vi "Configure Output Resistance.vi"(0 "VISA resource name":refnum<visa-resource-name>, 1 "List of Source Type":i32[](array[ring])=[1] items=["CURR", "VOLT"], 2 "Shunt Resistance Level (2E+9 Ohm)":dbl=2000000000.0, 3 "Enable Programmable Output (F: Disable)":bool, 5 "Output Channel (0: Channel 1)":i32(ring) items=["Channel 1", "Channel 2"], 7 "Source Mode (1: Voltage)":i32(ring)=1 items=["Current", "Voltage"], 9 "Operation Mode (0: Fixed)":i32(ring) items=["Fixed", "Emulate"], 11 "error in (no error)":errorcluster, 12 "List of Output Data":dbl[](array[numeric])=[0.0, 0.0], 13 "Series Resistance Level (0 Ohm)":dbl) -> (4 "VISA resource name out":refnum<visa-resource-name>, 15 "error out":errorcluster)   [LabVIEW 2023, in "Agilent B2900 Series.lvlib"]
doc: "Configure the output resistance.\n\n<B>Note:</B>\nThis VI is only supported by Agilent models B2961A, B2962A, B2961B and B2962B."
uses:
  Agilent B2900 Series.lvlib
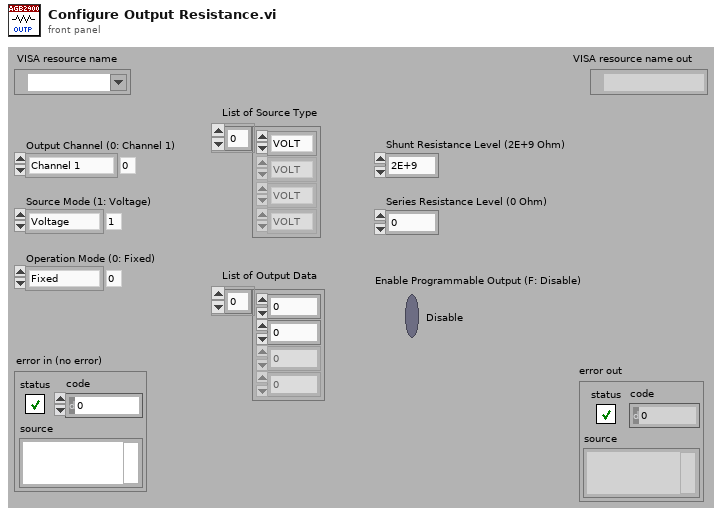
[diagram p1: front panel]
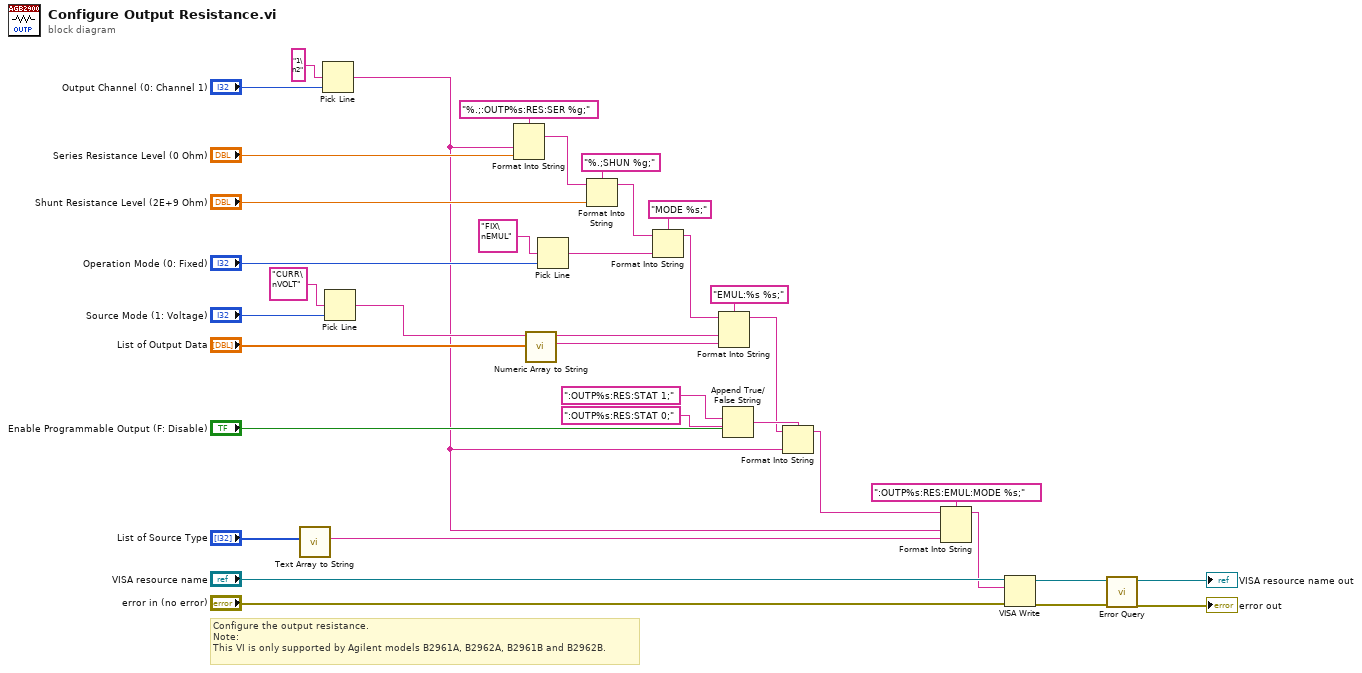
[diagram p0: block diagram]
diagram:
  # "Configure the output resistance.\nNote:\nThis VI is only supported by Agilent models B2961A, B2962A, B2961B and B2962B."
  n1 = call "Text Array to String.vi"("List Data"="List of Source Type") -> ("Result String"=w10:string)  [unwired: 10 in]
  n2 = Pick Line(multi-line string="1\n2", line index="Output Channel (0: Channel 1)") -> (output string=w6:string)  [unwired: 1 in]
  n3 = Pick Line(multi-line string="CURR\nVOLT", line index="Source Mode (1: Voltage)") -> (output string=w7:string)  [unwired: 1 in]
  n4 = Format Into String(format string="%.;:OUTP%s:RES:SER %g;", w6, "Series Resistance Level (0 Ohm)") -> (resulting string=w34:string)  [unwired: 2 in, 1 out]
  n5 = call "Numeric Array to String.vi"("List Data"="List of Output Data") -> ("Result String"=w14:string)  [unwired: 10 in]
  n6 = Pick Line(multi-line string="FIX\nEMUL", line index="Operation Mode (0: Fixed)") -> (output string=w18:string)  [unwired: 1 in]
  n7 = Format Into String(format string="%.;SHUN %g;", initial string=w34, "Shunt Resistance Level (2E+9 Ohm)") -> (resulting string=w17:string)  [unwired: 1 in, 1 out]
  n8 = Format Into String(format string="MODE %s;", initial string=w17, w18) -> (resulting string=w16:string)  [unwired: 1 in, 1 out]
  n9 = Format Into String(format string="EMUL:%s %s;", initial string=w16, w7, w14) -> (resulting string=w8:string)  [unwired: 1 in, 1 out]
  n10 = Append True/False String(1:"Enable Programmable Output (F: Disable)", 2:":OUTP%s:RES:STAT 0;", 3:":OUTP%s:RES:STAT 1;") -> (0:w11:string)  [unwired: 1 in]
  n11 = Format Into String(format string=w11, initial string=w8, w6) -> (resulting string=w9:string)  [unwired: 1 in, 1 out]
  n12 = Format Into String(format string=":OUTP%s:RES:EMUL:MODE %s;", initial string=w9, w6, w10) -> (resulting string=w1:string)  [unwired: 1 in, 1 out]
  n13 = VISA Write(VISA resource name="VISA resource name", write buffer=w1, error in (no error)="error in (no error)") -> (VISA resource name out=w5:refnum<visa-resource-name>, error out=w4:errorcluster)  [unwired: 1 out]
  n14 = call "Error Query.vi"("error in (no error)"=w4, "VISA resource name"=w5) -> ("error out"=→"error out":errorcluster, "VISA resource name out"=→"VISA resource name out":refnum<visa-resource-name>)  [unwired: 8 out]
